vi "getPayloadRequirement.vi"(11 "ControlPacket in":refnum<class "ControlPacket.lvclass">) -> (2 "Requirement":T1, 3 "ControlPacket out":refnum<class "ControlPacket.lvclass">)   [LabVIEW 2013, in "MQTT_Control_Packets.lvlib" / "ControlPacket.lvclass"]
uses:
  ControlPacket.lvclass
  Requirement -- enum.ctl
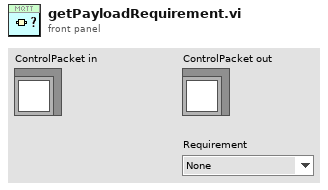
[diagram p1: front panel]
types:
  T1 = typedef "MQTT_Control_Packets.lvlib/ControlPacket.lvclass/Requirement -- enum.ctl" = enum16{"None", "Optional", "Required"}
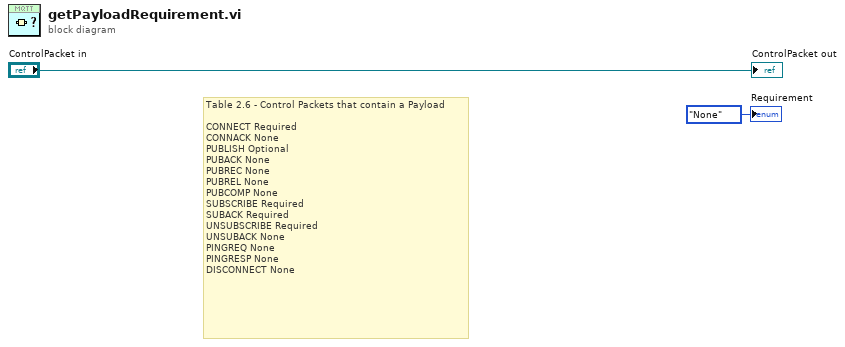
[diagram p0: block diagram]
diagram:
  # "Table 2.6 - Control Packets that contain a Payload\n\nCONNECT Required\nCONNACK None\nPUBLISH Optional\nPUBACK None\nPUBREC None\nPUBREL None\nPUBCOMP None\nSUBSCRIBE Required\nSUBACK Required\nUNSUBSCRIBE Required\nUNSUBACK None\nPINGREQ None\nPINGRESP None\nDISCONNECT None"
  "ControlPacket out" <- "ControlPacket in"
  "Requirement" <- Requirement_--_enum."None" ("Requirement")
